vi "OP300ZP_Vout.vi"(8 "errin":errorcluster caption="entrée d'erreur (pas d'erreur)", 11 "VISA":refnum<visa-resource-name> caption="Nom de ressource VISA") -> (0 "errout":errorcluster caption="sortie d'erreur", 3 "Vout lissée":dbl)   [LabVIEW 2020]
panel:
  out "read buffer":string
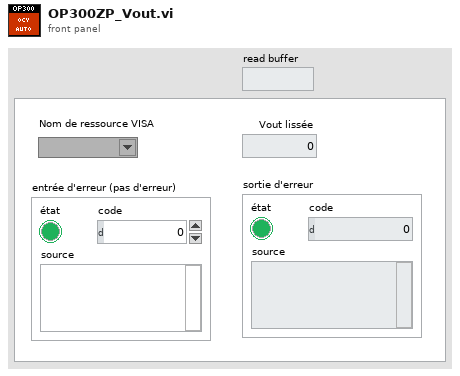
[diagram p1: front panel]
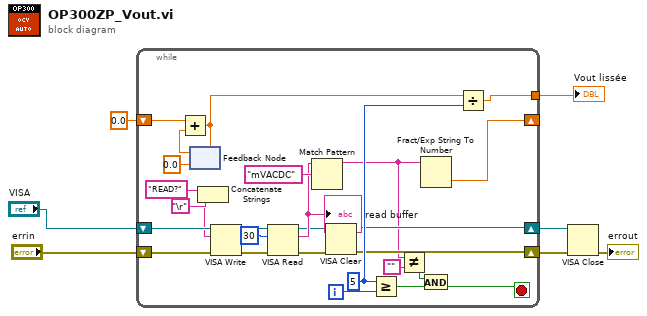
[diagram p0: block diagram]
diagram:
  n1 = while {
    shift-right: [w13] -> w6
    shift-left: "errin" -> [w34]
    shift-right: [w15] -> w5
    shift-left: "VISA" -> [w33]
    shift-right: [w22] -> _
    shift-left: 0.0 -> [w21]
    tunnel: [w17] -> w3
    i -> [w23]
    stop <- w11 stop-if-true
    w19 = 5 ("x")
    n2 = feedback #1(0.0) -> (w20:dbl)
    n3 = Add(x=w21, y=w20) -> (x+y=w18:dbl)
    n4 = feedback-in #1(w18) -> ()
    n5 = Concatenate Strings("READ?" ("chaîne"), "\r") -> (w27:string)
    n6 = VISA Write(VISA resource name=w33, write buffer=w27, error in (no error)=w34) -> (VISA resource name out=w29:refnum<visa-resource-name>, error out=w30:errorcluster)  [unwired: 1 out]
    n7 = VISA Read(VISA resource name=w29, byte count=u32 30 ("nombre d'octets"), error in (no error)=w30) -> (VISA resource name out=w16:refnum<visa-resource-name>, read buffer=w25:string, error out=w14:errorcluster)  [unwired: 1 out]
    "read buffer" <- w25
    n8 = Match Pattern(string=w25, regular expression="mVACDC" ("expression régulière")) -> (before substring=w8:string)  [unwired: 1 in, 3 out]
    n9 = VISA Clear(VISA resource name=w16, error in (no error)=w14) -> (VISA resource name out=w15:refnum<visa-resource-name>, error out=w13:errorcluster)
    n10 = Greater Or Equal?(x=w19, y=w23) -> (x >= y?=w24:bool)
    n11 = Not Equal?(x=w8, y="") -> (x != y?=w10:bool)
    n12 = Fract/Exp String To Number(string=w8) -> (number=w22:dbl)  [unwired: 3 in, 1 out]
    n13 = And(x=w10, y=w24) -> (x .and. y?=w11:bool)
    n14 = Divide(x=w18, y=w19) -> (x/y=w17:dbl)
  }
  "Vout lissée" <- w3
  n15 = VISA Close(VISA resource name=w5, error in (no error)=w6) -> (error out=→"errout":errorcluster)
